vi "PopupDebugProcess.vi"() -> ()   [LabVIEW 2011]
uses:
  Popup_ShowHideProcess.ctl
  100_PROCESS/SubVis/Enum_HideShow_Process.ctl
  030 - EVENTS/EnumFgvEventCommand.ctl
  090 - ERRORS/Ctrls/enumLogAndView.ctl
  100_PROCESS/SubVis/EnumFgvReferenceProcess.ctl
  030 - EVENTS/02 - ToScreens/ToScreensCommand.ctl
panel:
  out "Logo 600 X 200":picture
  in  "Array Show Hide Process":T1[](array[typedef])
  in  "StringParam":string
  in  "bouton_quitter":bool
  # "DEBUG process"
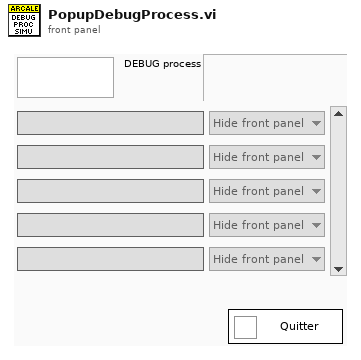
[diagram p1: front panel]
types:
  T1 = typedef "Popup_ShowHideProcess.ctl" = cluster{"Path":path, "VI Name":string, "Hide / Show":T2}
  T2 = typedef "Enum_HideShow_Process.ctl" = enum16{"Hide front panel", "Show front panel"}
  T3 = typedef "enumLogAndView.ctl" = enum16{"Log only", "Log and view"}
  T4 = typedef "EnumFgvEventCommand.ctl" = enum16{"Setup", "Cleanup", "Get"}
  T5 = typedef "EnumFgvReferenceProcess.ctl" = enum16{"Init", "Get", "Add Reference", "Close References"}
  T6 = typedef "ApplicationInfos.ctl" = cluster{"ApplicationName":string, "ApplicationVersion":string, "Logo 600X200 path":path, "Logo 400X400 path":path, "Client":string}
  T7 = typedef "ToScreensCommand.ctl" = enum16{"Stop screen", "Stop all screens"}
  T8 = enum32{"Invalid", "Standard", "Closed", "Hidden", "Minimized", "Maximized"}
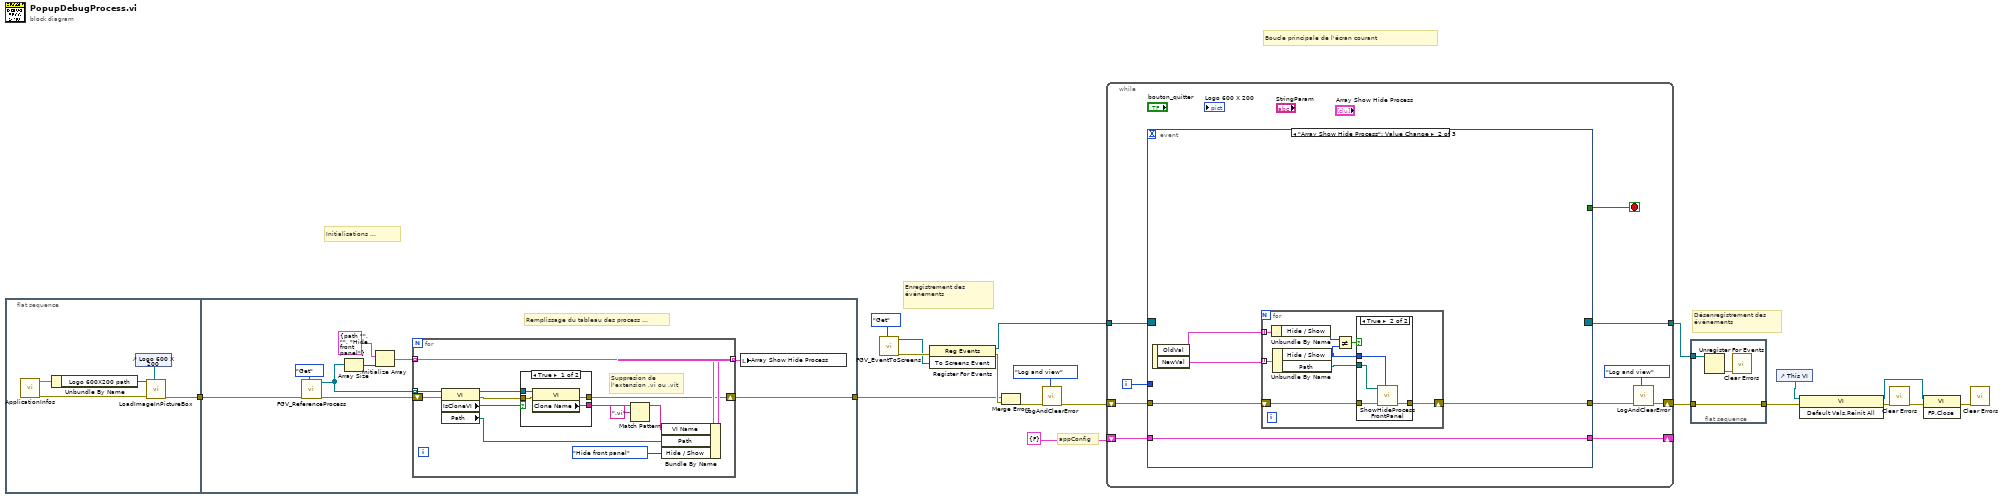
[diagram p0: block diagram]
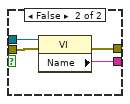
[diagram p2: hidden frame]
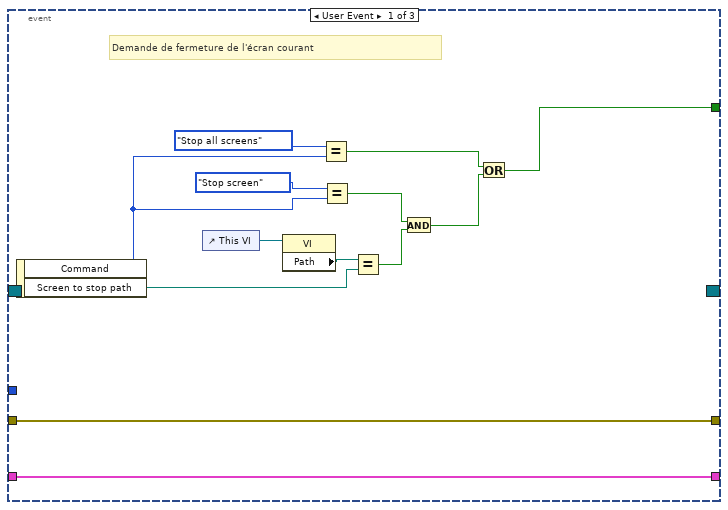
[diagram p3: hidden frame]
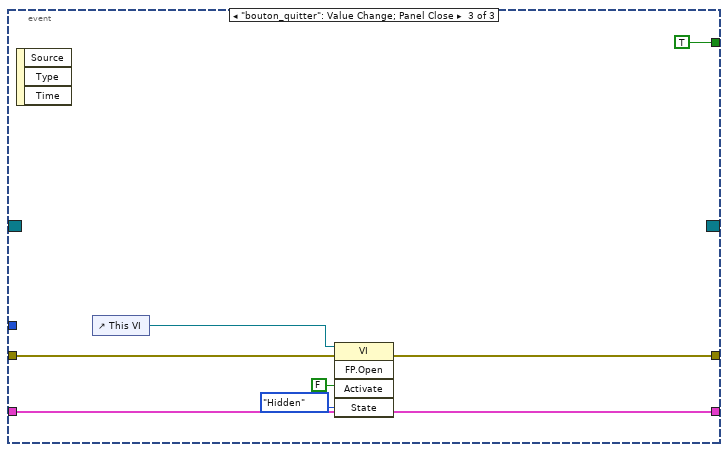
[diagram p5: hidden frame]
diagram:
  # "Initialisations ..."
  # "Boucle principale de l'écran courant"
  # "appConfig"
  # "Désenregistrement des \névénements"
  # "Enregistrement des \névénements"
  n1 = flat-sequence {
    tunnel: [w20] -> w8
    tunnel: w8 -> [w28]
    tunnel: [w32] -> w12
    frame #0 {
      n2 = call "ApplicationInfos.vi"() -> ("error out"=w24:errorcluster, "ApplicationInfo"=w22:T6)  [unwired: 10 in]
      n3 = Unbundle By Name(w22) -> ("Logo 600X200 path"=w21:path)
      n4 = control-ref of="Logo 600 X 200"() -> (w23:refnum<vi>)
      n5 = call "LoadImageInPictureBox.vi"("Pict Refnum In"=w23, "error in (no error)"=w24, "Image file path"=w21) -> ("error out"=w20:errorcluster)  [unwired: 8 in]
    }
    frame #1 {
      # "Remplissage du tableau des process ..."
      n6 = call "FGV_ReferenceProcess.vi"("Commande"=EnumFgvReferenceProcess."Get", "error in (no error)"=w28) -> ("error out"=w27:errorcluster, "ProcessReferences"=w26:refnum<vi>[])  [unwired: 8 in]
      n7 = Array Size(array=w26) -> (size(s)=w30:i32)
      n8 = Initialize Array(T1 {"Path"=path "", "VI Name"="", "Hide / Show"=enum."Hide front panel"}, w30) -> (w29:T1[])
      n9 = for {
        tunnel: [w45] -> w33 mode=indexing
        tunnel: w26 -> [w42] mode=indexing
        tunnel: w29 -> [w44] mode=indexing
        shift-right: [w37] -> w32
        shift-left: w27 -> [w43]
        # "Suppresion de l'extension .vi ou .vit"
        n10 = property class="VI"(reference=w42, error in=w43) -> (reference out=w39:refnum<vi>, error out=w38:errorcluster, "IsCloneVI"=w40:bool, "Path"=w41:path)
        n11 = case shown="True" w40 {
          tunnel: w39 -> [w50 w54]
          tunnel: w38 -> [w49 w53]
          tunnel: [w48 w52] -> w37
          tunnel: [w47 w51] -> w35
          frame True {
            n12 = property class="VI"(reference=w50, error in=w49) -> (error out=w48:errorcluster, "Clone Name"=w47:string)  [unwired: 1 out]
          }
          frame False {
            n13 = property class="VI"(reference=w54, error in=w53) -> (error out=w52:errorcluster, "Name"=w51:string)  [unwired: 1 out]
          }
        }
        n14 = Match Pattern(string=w35, regular expression=".vi") -> (before substring=w34:string)  [unwired: 1 in, 3 out]
        n15 = Bundle By Name(cluster=w44, "VI Name"=w34, "Path"=w41, "Hide / Show"=Enum_HideShow_Process."Hide front panel") -> (w45:T1)
      }
      n16 = local write "Array Show Hide Process"(w33) -> ()
    }
  }
  n17 = call "FGV_EventToScreens.vi"("Command"=EnumFgvEventCommand."Get") -> ("error out"=w16:errorcluster, "To Screens Event"=w14:refnum<user-event>)  [unwired: 9 in]
  n18 = register-events(error in=w16, w14) -> (reference out=w19:refnum<event-registration>, error out=w13:errorcluster)  [unwired: 1 in]
  n19 = Merge Errors(w12, w13) -> (w6:errorcluster)
  n20 = call "LogAndClearError.vi"("Log and view ?"=enumLogAndView."Log and view", "error in (no error)"=w6) -> ("error out"=w5:errorcluster)  [unwired: 9 in]
  n21 = while {
    tunnel: w19 -> [w64]
    shift-right: [w56] -> w11
    shift-left: w5 -> [w63]
    tunnel: [w62] -> w9
    shift-right: [w60] -> _
    shift-left: cluster{"Boolean":bool} {"Boolean"=FALSE} ("appConfig") -> [w61]
    i -> [w58]
    stop <- w59 stop-if-true
    n22 = event shown="[1] \"Array Show Hide Process\": Value Change" {
      selector: w64 -> [_ _ _]
      dyn-events: [_ _ _] -> w62
      timeout: _ -> [_ _ _]
      tunnel: [w66 _ TRUE ("stopCurrentScreen")] -> w59
      tunnel: w63 -> [w65 w80 w100]
      tunnel: [w65 w79 w99] -> w57
      tunnel: w61 -> [w77 w82 w101]
      tunnel: [w77 w82 w101] -> w60
      tunnel: w58 -> [_ _ _]
      event User Event {
        # "Demande de fermeture de l'écran courant"
        n23 = event-data() -> ("Command"=w74:T7, "Screen to stop path"=w71:path)  [unwired: 1 out]
        n24 = control-ref of="This VI"() -> (w73:refnum<vi>)
        n25 = property class="VI"(reference=w73) -> ("Path"=w72:path)  [unwired: 1 in, 2 out]
        n26 = Equal?(x=ToScreensCommand."Stop all screens", y=w74) -> (x = y?=w68:bool)
        n27 = Equal?(x=ToScreensCommand."Stop screen", y=w74) -> (x = y?=w70:bool)
        n28 = Equal?(x=w72, y=w71) -> (x = y?=w69:bool)
        n29 = And(x=w70, y=w69) -> (x .and. y?=w67:bool)
        n30 = Or(x=w68, y=w67) -> (x .or. y?=w66:bool)
      }
      event "Array Show Hide Process": Value Change {
        n31 = event-data() -> ("OldVal"=w78:T1[], "NewVal"=w81:T1[])  [unwired: 1 out]
        n32 = for {
          tunnel: w81 -> [w88] mode=indexing
          shift-right: [w89] -> w79
          shift-left: w80 -> [w90]
          tunnel: w78 -> [w86] mode=indexing
          n33 = Unbundle By Name(w86) -> ("Hide / Show"=w84:T2)
          n34 = Unbundle By Name(w88) -> ("Hide / Show"=w85:T2, "Path"=w87:path)
          n35 = Not Equal?(x=w84, y=w85) -> (x != y?=w83:bool)
          n36 = case shown="True" w83 {
            tunnel: w90 -> [w91 w95]
            tunnel: [w91 w92] -> w89
            tunnel: w87 -> [_ w94]
            tunnel: w85 -> [_ w93]
            frame False {
            }
            frame True {
              n37 = call "ShowHideProcessFrontPanel.vi"("Hide / Show front panel"=w93, "error in (no error)"=w95, "Process path"=w94) -> ("error out"=w92:errorcluster)  [unwired: 8 in]
            }
          }
        }
      }
      event "bouton_quitter": Value Change; Panel Close {
        n38 = event-data() -> ()  [unwired: 4 out]
        n39 = control-ref of="This VI"() -> (w98:refnum<vi>)
        n40 = invoke class="VI" method="FP.Open"(reference=w98, error in=w100, "Activate"=FALSE ("Activate?"), "State"=T8."Hidden") -> (error out=w99:errorcluster)  [unwired: 1 in, 4 out]
      }
    }
    n41 = call "LogAndClearError.vi"("Log and view ?"=enumLogAndView."Log and view", "error in (no error)"=w57) -> ("error out"=w56:errorcluster)  [unwired: 9 in]
  }
  n42 = flat-sequence {
    tunnel: w9 -> [w105]
    tunnel: w11 -> [w103]
    tunnel: [w103] -> w10
    frame #0 {
      n43 = Unregister For Events(event registration refnum=w105) -> (error out=w104:errorcluster)  [unwired: 1 in]
      n44 = call <vilib>:"Clear Errors.vi"("error in (no error)"=w104) -> ()  [unwired: 7 out]
    }
  }
  n45 = control-ref of="This VI"() -> (w1:refnum<vi>)
  n46 = invoke class="VI" method="Default Vals.Reinit All"(reference=w1, error in=w10) -> (reference out=w2:refnum<vi>, error out=w17:errorcluster)  [unwired: 1 in, 1 out]
  n47 = call <vilib>:"Clear Errors.vi"("error in (no error)"=w17) -> ("error out"=w3:errorcluster)  [unwired: 6 out]
  n48 = invoke class="VI" method="FP.Close"(reference=w2, error in=w3) -> (error out=w4:errorcluster)  [unwired: 1 in, 2 out]
  n49 = call <vilib>:"Clear Errors.vi"("error in (no error)"=w4) -> ()  [unwired: 7 out]
